vi "combined arm safety.vi"(7 "Input":dbl) -> (8 "Safe Output":dbl, 13 "Safety Data":T1)   [LabVIEW 2013]
uses:
  typedefs/Dashboard/dashboard safety status data.ctl
  typedefs/fg_typedef.ctl
  typedefs/DevRef Type.ctl
  typedefs/State Machine/subStates.ctl
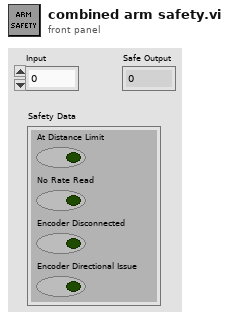
[diagram p1: front panel]
types:
  T1 = typedef "dashboard safety status data.ctl" = cluster{"At Distance Limit":bool, "No Rate Read":bool, "Encoder Disconnected":bool, "Encoder Directional Issue":bool}
  T2 = typedef "subStates.ctl" = enum16{"null", "wait", "driver control", "auto", "manual override", "hold position", "rotate", "pickup", "pass", "recover pass", "load", "goto shoot", "shoot high goal", "shoot low goal", "cancel arm", "cancel shooter", "end", "test"}
  T3 = typedef "DevRef Type.ctl" = enum16{"Shooter Solenoid", "Latch Solenoid", "Right Up Sensor", "Right Down Sensor", "Hold Sensor", "2 Ball Switch", "Arm Encoder"}
  T4 = typedef "fg_typedef.ctl" = enum16{"Get", "Set"}
  T5 = typedef "WPI_EncoderDevRef.ctl" = cluster{"DevStatus":errorcluster, "EncoderIndex":T6, "CounterIndex":T7, "DistancePerCount":dbl, "Decoding Type":T8}
  T6 = typedef "FPGA_EncoderIdx.ctl" = enum8{"Enc 0", "Enc 1", "Enc 2", "Enc 3", "Invalid"}
  T7 = typedef "FPGA_CounterCtrSystemIndex.ctl" = enum8{"Ctr 0", "Ctr 1", "Ctr 2", "Ctr 3", "Ctr 4", "Ctr 5", "Ctr 6", "Ctr 7", "Invalid"}
  T8 = typedef "WPI_EncoderType.ctl" = enum16{"1x", "2x", "4x"}
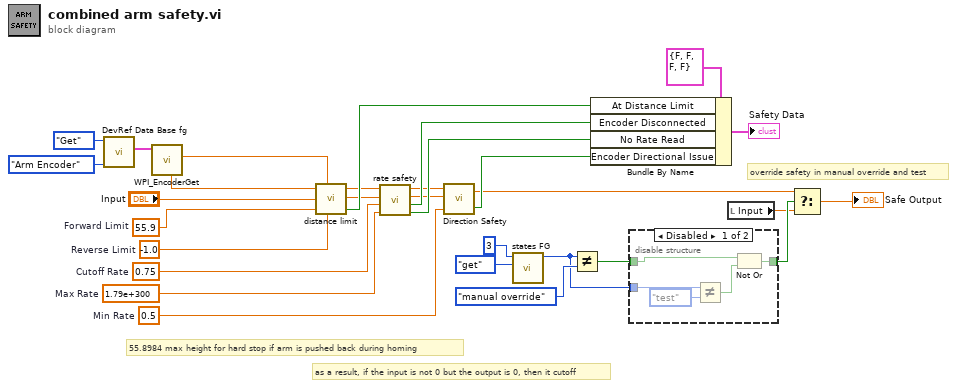
[diagram p0: block diagram]
diagram:
  w24 = 1.79e+300  # Max Rate
  w23 = 0.5  # Min Rate
  w2 = 0.75  # Cutoff Rate
  w25 = -1.0  # Reverse Limit
  w26 = 55.9  # Forward Limit
  # "override safety in manual override and test"
  # "55.8984 max height for hard stop if arm is pushed back during homing"
  # "as a result, if the input is not 0 but the output is 0, then it cutoff"
  n1 = call "DevRef Data Base fg.vi"("DevRef to Get"=DevRef_Type."Arm Encoder", "Menu"=fg_typedef."Get") -> ("Selected Encoder"=w29:T5)  [unwired: 2 in, 5 out]
  n2 = call <vilib>:"WPI_EncoderGet.vi"("EncoderDevRef"=w29) -> ("Distance"=w27:dbl, "Rate"=w28:dbl)  [unwired: 5 in, 4 out]
  n3 = call "distance limit.vi"("Encoder Rate"=w28, "Encoder Distance"=w27, "Desired Rate"="Input", "Forward Limit"=w26, "Reverse Limit"=w25) -> ("Encoder Rate Out"=w13:dbl, "Output Rate"=w1:dbl, "At Distance Limit"=w17:bool)
  n4 = call "rate safety.vi"("Max Rate"=w24, "Cutoff Rate"=w2, "Desired Rate"=w1, "Encoder Rate"=w13) -> ("No Rate Read"=w15:bool, "Encoder Disconnected"=w16:bool, "Output Rate"=w11:dbl, "Encoder Rate Out"=w12:dbl)
  n5 = call "Direction Safety.vi"("Min Rate"=w23, "Desired Rate"=w11, "Encoder Rate"=w12) -> ("Encoder Directional Issue"=w14:bool, "Super Safe Rate"=w9:dbl)
  n6 = call "states FG.vi"("menu (get)"=enum16{"set", "get"}."get", "Loop ID"=3) -> ("subState out"=w6:T2)  [unwired: 6 in, 3 out]
  n7 = Not Equal?(x=w6, y=subStates."manual override") -> (x != y?=w5:bool)
  n8 = Bundle By Name(cluster=T1 {"At Distance Limit"=FALSE, "No Rate Read"=FALSE, "Encoder Disconnected"=FALSE, "Encoder Directional Issue"=FALSE} ("Input"), "At Distance Limit"=w17, "Encoder Disconnected"=w16, "No Rate Read"=w15, "Encoder Directional Issue"=w14) -> (→"Safety Data":T1)
  n9 = disable-structure shown="Disabled" {
    disable-tunnel: w6 -> [w35 _]
    disable-tunnel: w5 -> [w33 w36]
    disable-tunnel: [w31 w36] -> w4
    frame Disabled {
      n10 = Not Equal?(x=w35, y=subStates."test") -> (x != y?=w32:bool)
      n11 = Not Or(1:w32, 2:w33) -> (0:w31:bool)
    }
    frame Enabled {
    }
  }
  n12 = local read "Input"() -> (w3:dbl)
  n13 = Select(t=w9, s=w4, f=w3) -> (s? t:f=→"Safe Output":dbl)
